vi "CpuLoadsNTServer.vi"() -> ()   [LabVIEW 2019]
doc: "This VI implements the framework and scheduler for your robotics program. It should not be necessary to modify the framework. You are expected to add your code to the VIs called from Robot Main - the ones located in the Team Code folder within the project."
uses:
  <vilib>/NI_Real-Time Target Support.lvlib
panel:
  out "IndividualCpuLoads":dbl[](array[numeric]) format="%11.2f"
  out "Cpu Loads":dbl format="%11.2f"
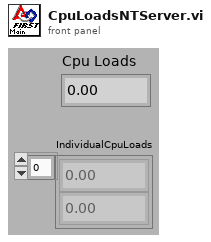
[diagram p1: front panel]
types:
  T1 = typedef "NI_Real-Time Target Support.lvlib/RT CPU Load.ctl" = cluster{"Total (%)":dbl, "Time Critical (%)":dbl, "Timed Structures (%)":dbl, "High (%)":dbl, "Above Normal (%)":dbl, "Normal (%)":dbl, "Background (%)":dbl, "Idle (%)":dbl, "ISR (%)":dbl}
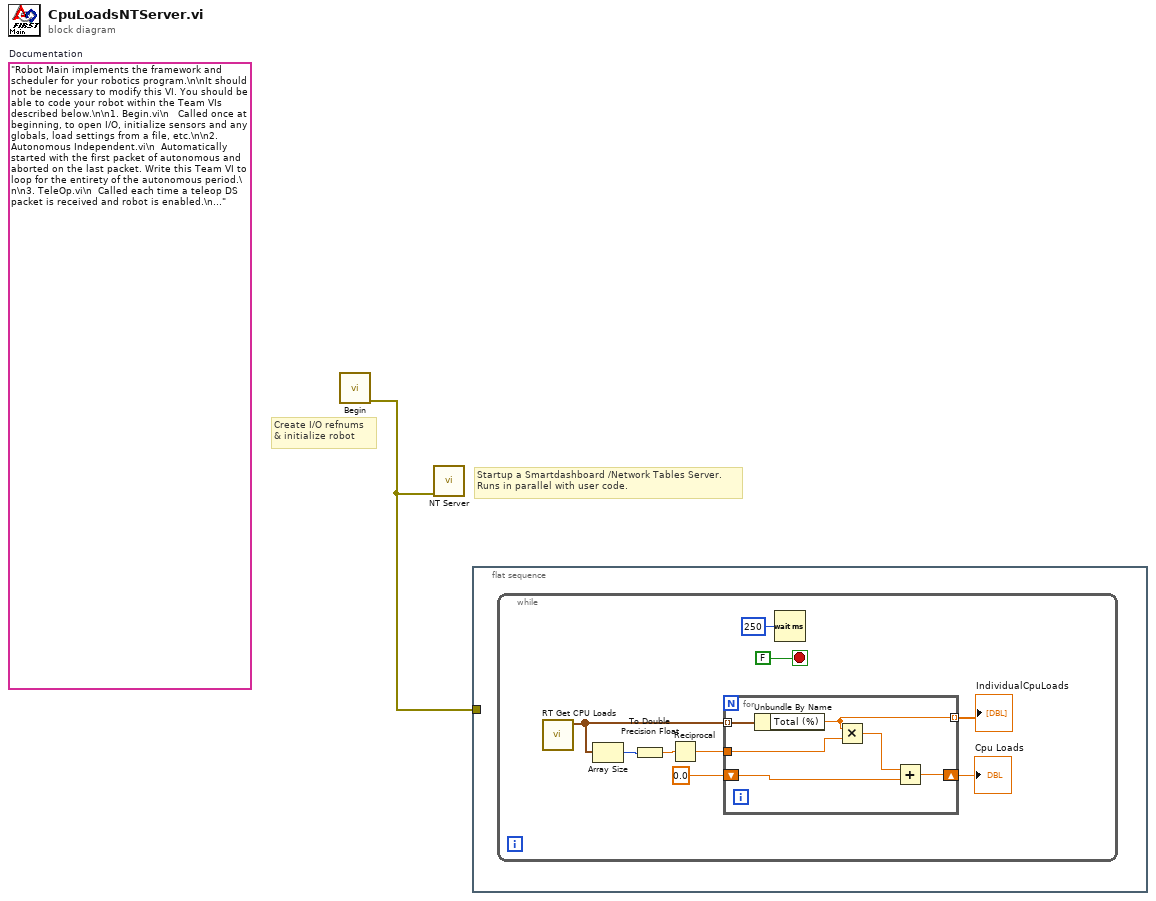
[diagram p0: block diagram]
diagram:
  (unwired) "Robot Main implements the framework and scheduler for your robotics program.\n\nIt should not be necessary to modify this VI. You should be able to code your robot within the Team VIs described below.\n\n1. Begin.vi\n   Called once at beginning, to open I/O, initialize sensors and any globals, load settings from a file, etc.\n\n2. Autonomous Independent.vi\n  Automatically started with the first packet of autonomous and aborted on the last packet. Write this Team VI to loop for the entirety of the autonomous period.\n\n3. TeleOp.vi\n  Called each time a teleop DS packet is received and robot is enabled.\n\n4. Disabled.vi\n  Called each time a packet is received and the robot is disabled.\n\n5. Test.vi\n  Called Automatically started with the first test packet and aborted on the last. Modify this VI to carry out robot and sensor validation tests.\n\n6. Vision Processing.vi\n  A parallel loop that acquires and processes camera images. Drag from the project/Team Code if you wish to use this.\n\n7. PeriodicTasks.vi\n  Parallel loops running at user-defined rates.\n\n8. Finish.vi\n  Called before exiting, so you can save data, clean up I/O, etc.\n"  # Documentation
  # "Startup a Smartdashboard /Network Tables Server.\nRuns in parallel with user code."
  # "Create I/O refnums\n& initialize robot"
  n1 = call "Begin.vi"() -> ("error out"=w1:errorcluster)  [unwired: 2 in, 9 out]
  n2 = call <vilib>:"NT Server.vi"("error in (no error)"=w1) -> ()  [unwired: 11 in]
  n3 = flat-sequence {
    tunnel: w1 -> [_]
    frame #0 {
      n4 = while {
        stop <- FALSE stop-if-true
        n5 = call <vilib>:"RT Get CPU Loads.vi"() -> ("CPU loads"=w8:T1[])  [unwired: 10 in, 1 out]
        n6 = Array Size(array=w8) -> (size(s)=w7:i32)
        n7 = To Double Precision Float(number=w7) -> (double precision float=w6:dbl)
        n8 = Reciprocal(x=w6) -> (1/x=w5:dbl)
        n9 = for {
          tunnel: w8 -> [w16] mode=indexing
          tunnel: w5 -> [w15]
          shift-right: [w12] -> w2
          shift-left: 0.0 -> [w14]
          tunnel: [w11] -> w3 mode=indexing
          n10 = Unbundle By Name(w16) -> ("Total (%)"=w11:dbl)
          n11 = Multiply(x=w11, y=w15) -> (x*y=w13:dbl)
          n12 = Add(x=w13, y=w14) -> (x+y=w12:dbl)
        }
        "IndividualCpuLoads" <- w3
        "Cpu Loads" <- w2
        n13 = Wait (ms)(milliseconds to wait=u32 250) -> ()  [unwired: 1 out]
      }
    }
  }
